vi "Digitalizer.vi"(0 "Analog_Waveform":waveform(dbl), 5 "Amplitude (V)":dbl) -> (4 "Digital_Waveform":digitaldata)   [LabVIEW 2023]
doc: "This VI digitalize the analog waveform."
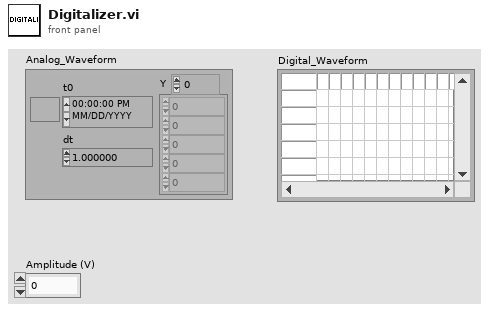
[diagram p1: front panel]
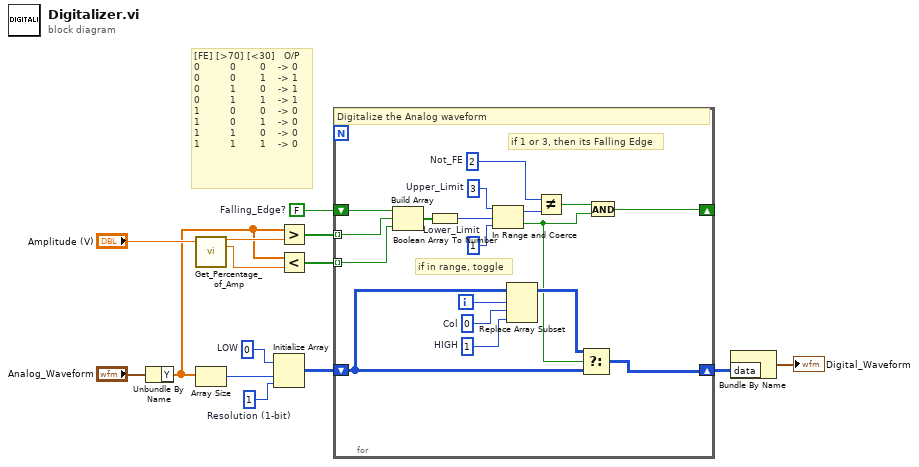
[diagram p0: block diagram]
diagram:
  w1 = 1  # Resolution (1-bit)
  w12 = FALSE  # Falling_Edge?
  w13 = u8 0  # LOW
  # "[FE] [>70] [<30]   O/P    \n0          0        0    -> 0 \n0          0        1    -> 1    \n0          1        0    -> 1    \n0          1        1    -> 1\n1          0        0    -> 0 \n1          0        1    -> 0\n1          1        0    -> 0\n1          1        1    -> 0"
  n1 = Unbundle By Name ("Get Waveform Components")("Analog_Waveform") -> ("Y"=w4:dbl[])
  n2 = call "Get_Percentage_of_Amp.vi"("Amplitude(V)"="Amplitude (V)") -> ("End_Point"=w6:dbl, "Start_Point"=w7:dbl)  [unwired: 12 in, 1 out]
  n3 = Array Size(array=w4) -> (size(s)=w10:i32)
  n4 = Initialize Array(w13, w10, w1) -> (w14:u8[][])
  n5 = Greater?(x=w4, y=w6) -> (0:w3:bool[])
  n6 = Less?(x=w4, y=w7) -> (x < y?=w2:bool[])
  n7 = for {
    shift-right: [w15] -> _
    shift-left: w12 -> [w31]
    shift-right: [w17] -> w8
    shift-left: w14 -> [w19]
    tunnel: w3 -> [w30] mode=indexing
    tunnel: w2 -> [w29] mode=indexing
    i -> [w28]
    w21 = u32 2  # Not_FE
    w24 = u32 1  # Lower_Limit
    w23 = u32 3  # Upper_Limit
    w27 = 0  # Col
    w26 = u8 1  # HIGH
    # "if in range, toggle"
    # "if 1 or 3, then its Falling Edge"
    # "Digitalize the Analog waveform"
    n8 = Build Array(w31, w30, w29) -> (w32:bool[])
    n9 = Boolean Array To Number(Boolean array=w32) -> (number=w25:u32)
    n10 = In Range and Coerce(upper limit=w23, x=w25, lower limit=w24) -> (coerced(x)=w22:u32, In Range?=w16:bool)
    n11 = Replace Array Subset(array=w19, new element=w26, index (row)=w28, index (col)=w27) -> (w18:u8[][])
    n12 = Not Equal?(x=w21, y=w22) -> (x != y?=w20:bool)
    n13 = Select(t=w18, s=w16, f=w19) -> (s? t:f=w17:u8[][])
    n14 = And(x=w20, y=w16) -> (x .and. y?=w15:bool)
  }
  n15 = Bundle By Name("data"=w8) -> (→"Digital_Waveform":digitaldata)  [unwired: 1 in]
